vi "sub_Parse_PCM_Frame.vi"(0 "In Buffer":string, 1 "每帧点数N":i32) -> (14 "Out Buffer":string, 15 "valid？":bool, 16 "Samples  I16":i16[](array[numeric]), 17 "Frame Length":u32, 18 "Parse Status":string)   [LabVIEW 2026]
panel:
  # "解析完一帧后剩下的缓存"
  # "输入串口缓存区内容"
  # "这次是否成功解析出一帧"
  # "一帧有多少个采样点"
  # "解析出来的 PCM 数组"
  # "当前解析出来的帧点数"
  # "返回状态文字，比如：\n未找到帧头\n数据不足一帧\n帧尾错误\n解析成功"
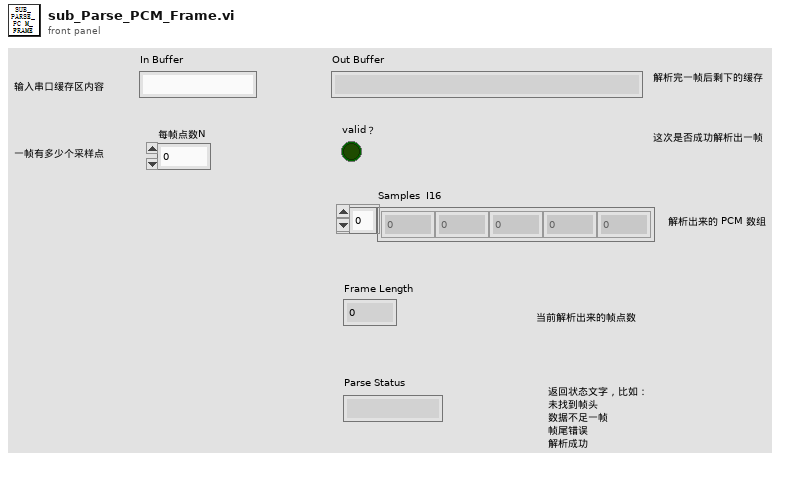
[diagram p1: front panel]
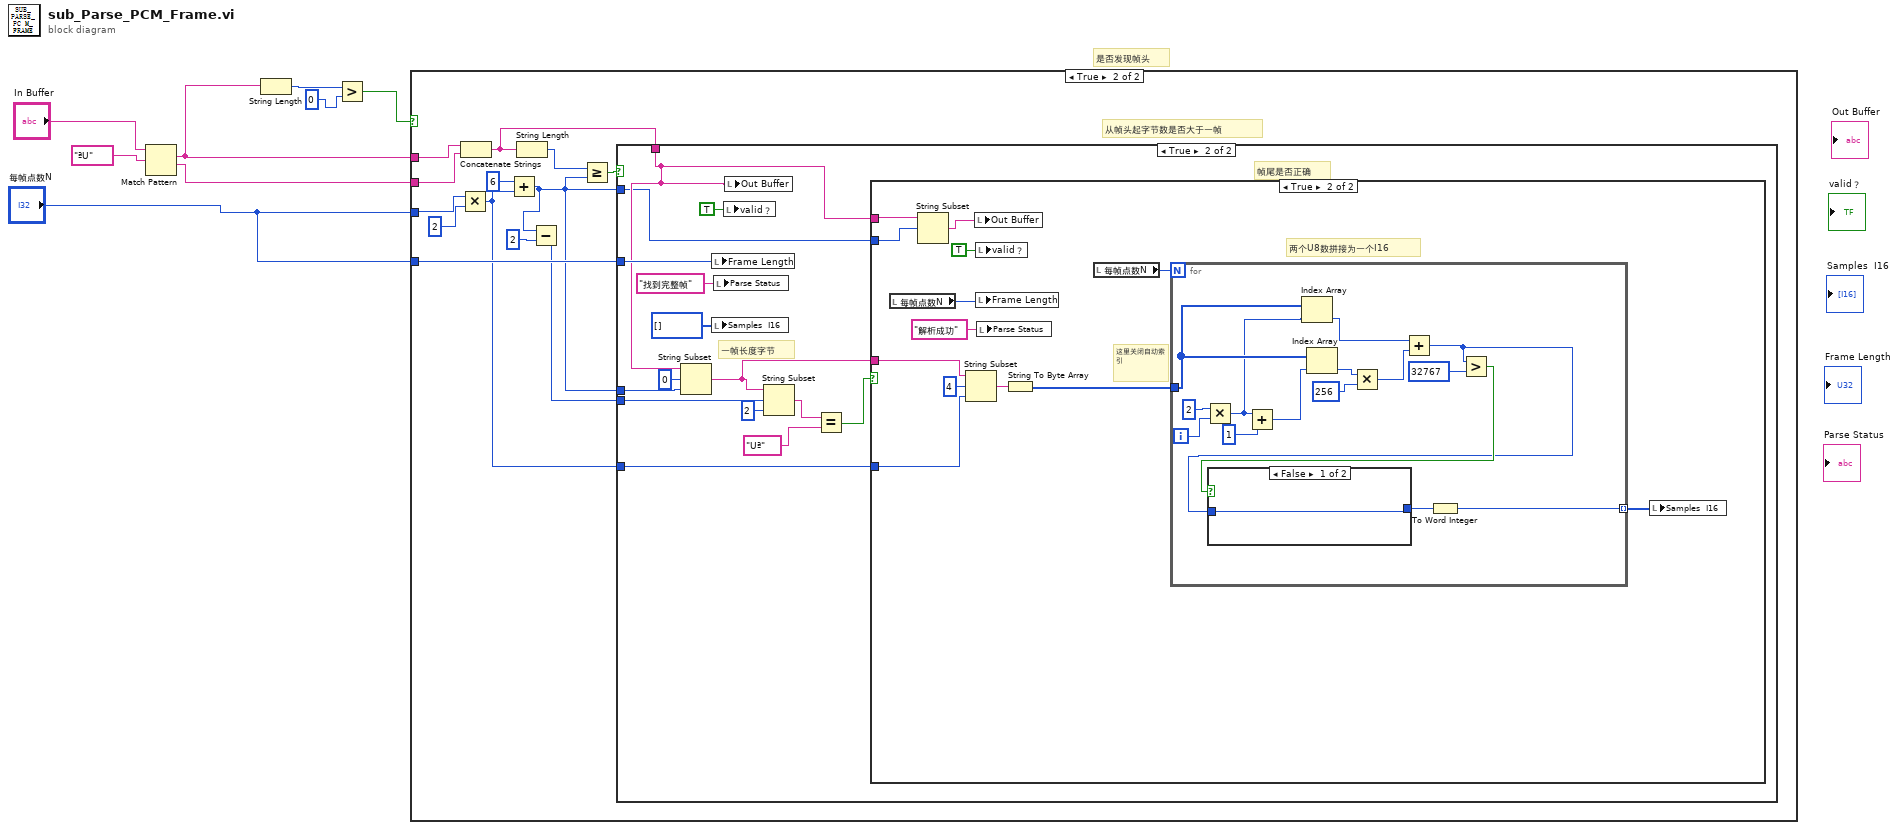
[diagram p0: block diagram]
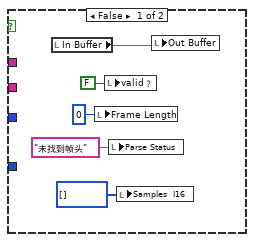
[diagram p2: hidden frame]
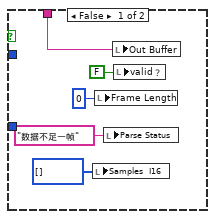
[diagram p3: hidden frame]
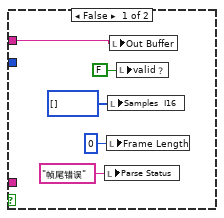
[diagram p4: hidden frame]
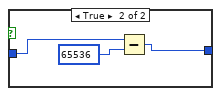
[diagram p5: hidden frame]
diagram:
  # "是否发现帧头"
  n1 = Match Pattern(string="In Buffer", regular expression="ªU") -> (match substring=w4:string, after substring=w3:string)  [unwired: 1 in, 2 out]
  n2 = String Length(string=w4) -> (length=w7:i32)
  n3 = Greater?(x=w7, y=0) -> (0:w6:bool)
  n4 = case shown="True" w6 {
    tunnel: "每帧点数N" -> [_ w26]
    tunnel: w4 -> [_ w23]
    tunnel: w3 -> [_ w22]
    tunnel: "每帧点数N" -> [_ w18]
    frame False {
      n5 = local read "In Buffer"() -> (w9:string)
      n6 = local write "Frame Length"(u32 0 ("Frame Length")) -> ()
      n7 = local write "valid？"(FALSE ("valid？")) -> ()
      n8 = local write "Parse Status"("未找到帧头" ("Parse Status")) -> ()
      n9 = local write "Samples  I16"(i16[] [] ("Samples  I16")) -> ()
      n10 = local write "Out Buffer"(w9) -> ()
    }
    frame True {
      # "从帧头起字节数是否大于一帧"
      n11 = Multiply(x=w26, y=2) -> (x*y=w15:i32)
      n12 = Concatenate Strings(w23, w22) -> (w19:string)
      n13 = Add(x=6, y=w15) -> (x+y=w14:i32)
      n14 = String Length(string=w19) -> (length=w21:i32)
      n15 = Subtract(x=w14, y=2) -> (x-y=w16:i32)
      n16 = Greater Or Equal?(x=w21, y=w14) -> (x >= y?=w20:bool)
      n17 = case shown="True" w20 {
        tunnel: w19 -> [w31 w35]
        tunnel: w18 -> [_ w45]
        tunnel: w14 -> [_ w41]
        tunnel: w16 -> [_ w40]
        tunnel: w15 -> [_ w33]
        tunnel: w14 -> [_ w32]
        frame False {
          n18 = local write "Samples  I16"(i16[] [] ("Samples  I16")) -> ()
          n19 = local write "Frame Length"(u32 0 ("Frame Length")) -> ()
          n20 = local write "Parse Status"("数据不足一帧" ("Parse Status")) -> ()
          n21 = local write "Out Buffer"(w31) -> ()
          n22 = local write "valid？"(FALSE ("valid？")) -> ()
        }
        frame True {
          # "帧尾是否正确"
          # "一帧长度字节"
          n23 = String Subset(string=w35, offset (0)=0, length (rest)=w41) -> (substring=w34:string)
          n24 = local write "Frame Length"(w45) -> ()
          n25 = local write "Samples  I16"(i16[] [] ("Samples  I16")) -> ()
          n26 = local write "Parse Status"("找到完整帧" ("Parse Status")) -> ()
          n27 = local write "valid？"(TRUE ("valid？")) -> ()
          n28 = local write "Out Buffer"(w35) -> ()
          n29 = String Subset(string=w34, offset (0)=w40, length (rest)=2 ("length (rest)")) -> (substring=w38:string)
          n30 = Equal?(x=w38, y="Uª") -> (x = y?=w36:bool)
          n31 = case shown="True" w36 {
            tunnel: w35 -> [w51 w54]
            tunnel: w34 -> [_ w61]
            tunnel: w33 -> [_ w59]
            tunnel: w32 -> [_ w53]
            frame False {
              n32 = local write "Parse Status"("帧尾错误" ("Parse Status")) -> ()
              n33 = local write "Frame Length"(u32 0 ("Frame Length")) -> ()
              n34 = local write "Samples  I16"(i16[] [] ("Samples  I16")) -> ()
              n35 = local write "Out Buffer"(w51) -> ()
              n36 = local write "valid？"(FALSE ("valid？")) -> ()
            }
            frame True {
              # "两个U8数拼接为一个I16"
              # "这里关闭自动索引"
              n37 = local read "每帧点数N"() -> (w63:i32)
              n38 = String Subset(string=w54, offset (0)=w53) -> (substring=w52:string)  [unwired: 1 in]
              n39 = String Subset(string=w61, offset (0)=4, length (rest)=w59) -> (substring=w58:string)
              n40 = local write "Out Buffer"(w52) -> ()
              n41 = local write "valid？"(TRUE ("valid？")) -> ()
              n42 = local write "Frame Length"(w63) -> ()
              n43 = local write "Parse Status"("解析成功" ("Parse Status")) -> ()
              n44 = String To Byte Array(string=w58) -> (unsigned byte array=w56:u8[])
              n45 = local read "每帧点数N"() -> (w57:i32)
              n46 = for {
                N: w57 -> [_]
                tunnel: w56 -> [w76]
                tunnel: [w65] -> w55 mode=indexing
                i -> [w78]
                n47 = Multiply(x=2, y=w78) -> (x*y=w75:i32)
                n48 = Add(x=w75, y=1) -> (x+y=w74:i32)
                n49 = Index Array(array=w76, index=w75) -> (element=w71:u8)
                n50 = Index Array(array=w76, index=w74) -> (element=w70:u8)
                n51 = Multiply(x=w70, y=256) -> (x*y=w72:i32)
                n52 = Add(x=w71, y=w72) -> (x+y=w67:i32)
                n53 = Greater?(x=w67, y=32767) -> (0:w68:bool)
                n54 = case shown="False" w68 {
                  tunnel: w67 -> [w80 w83]
                  tunnel: [w80 w81] -> w66
                  frame False {
                  }
                  frame True {
                    n55 = Subtract(x=w83, y=65536) -> (x-y=w81:i32)
                  }
                }
                n56 = To Word Integer(number=w66) -> (16bit integer=w65:i16)
              }
              n57 = local write "Samples  I16"(w55) -> ()
            }
          }
        }
      }
    }
  }
